vi "Compute Max Level.vi"(0 "FM Sweep in":refnum<class "FM Sweep.lvclass">, 1 "Filter in":refnum<class "Filter.lvclass">, 5 "Level in":refnum<class "Level.lvclass">, 7 "Fs (Hz)":dbl, 9 "Vmax":dbl, 11 "error in (no error)":errorcluster) -> (4 "FM Sweep out":refnum<class "FM Sweep.lvclass">, 6 "Level thru":refnum<class "Level.lvclass">, 10 "Lmax":dbl, 15 "error out":errorcluster)   [LabVIEW 2020, in "FM Sweep.lvclass"]
uses:
  FM Sweep.lvclass
  D:/Experiment VIs/Koop/KObject Class/KObject.lvclass
  Level/Level.lvclass
  Filter/Filter.lvclass
  FM Sweep.lvclass/FM Sweep.ctl
  Level/Level.lvclass/Level.ctl
  <vilib>/Analysis/baseanly.llb/Mean (DBL).vi
  Level/Read Units.vi
  Utility VIs/Math VIs/Linear to dB (scalar).vi
  <vilib>/Analysis/NI_AALBase.lvlib
  Koop/KObject Class/KObject.lvclass
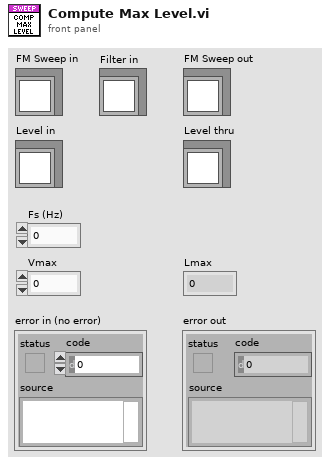
[diagram p1: front panel]
types:
  T1 = typedef "Level.lvclass/LevelUnits.ctl" = enum16{"dB atten", "dB SPL", "dB Vrms", "Volts", "dB mW", "mW", "dB HL", "dB SL"}
  T2 = cluster{"Freq (Hz)":dbl[], "Mag (dB SPL)":dbl[], "Phase (deg)":dbl[]}
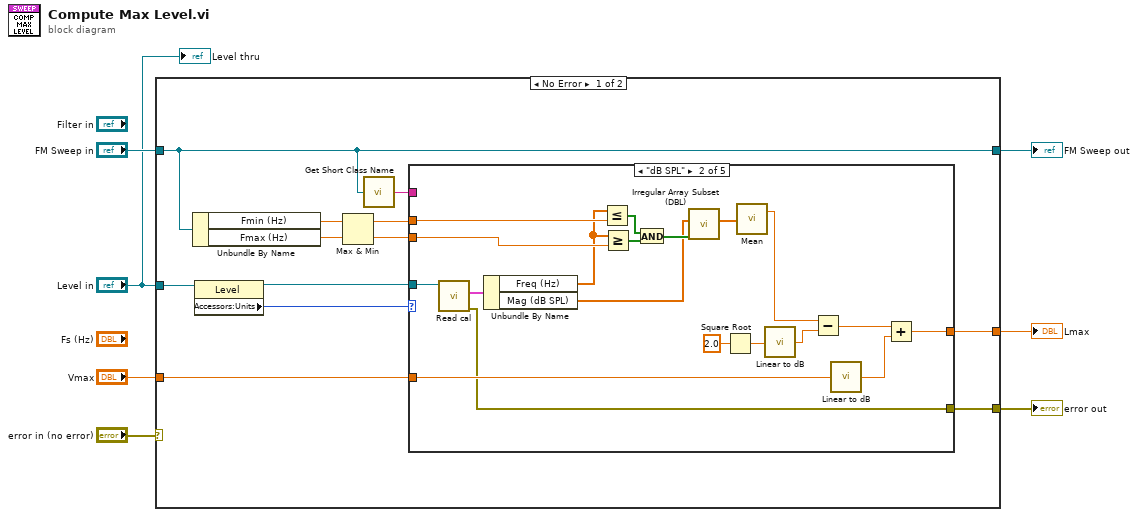
[diagram p0: block diagram]
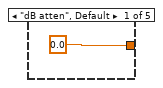
[diagram p2: hidden frame]
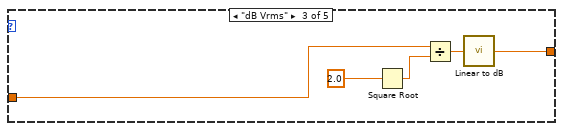
[diagram p3: hidden frame]
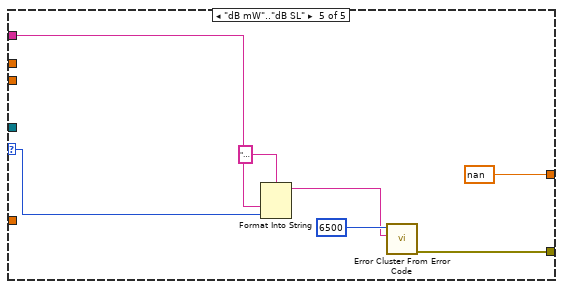
[diagram p5: hidden frame]
diagram:
  n1 = case shown="No Error" "error in (no error)" {
    selector: "error in (no error)" -> [_ w53]
    tunnel: "FM Sweep in" -> [w14 w54]
    tunnel: [w14 w54] -> w6
    tunnel: "Level in" -> [w19 _]
    tunnel: "Vmax" -> [w17 _]
    tunnel: [w16 _] -> w3
    tunnel: [w15 w53] -> w2
    frame No Error {
      n2 = Unbundle By Name(w14) -> ("Fmin (Hz)"=w11:dbl, "Fmax (Hz)"=w10:dbl)
      n3 = property class="Level"(reference=w19) -> (reference out=w12:refnum<class "Level.lvclass">, "Accessors:Units"=w18:T1)  [unwired: 1 in, 1 out]
      n4 = Max & Min(x=w11, y=w10) -> (max(x,y)=w9:dbl, min(x,y)=w8:dbl)
      n5 = call "Get Short Class Name.vi"("KObject in"=w14) -> ("Class"=w13:string)  [unwired: 4 in]
      n6 = case shown="\"dB SPL\"" w18 {
        selector: w18 -> [_ _ _ _ w47]
        tunnel: [0.0 ("Reference Level") w39 w41 w45 nan ("Vmax")] -> w16
        tunnel: [_ w21 _ _ w49] -> w15
        tunnel: w9 -> [_ w28 _ _ _]
        tunnel: w8 -> [_ w27 _ _ _]
        tunnel: w17 -> [_ w26 w40 w45 _]
        tunnel: w13 -> [_ _ _ _ w46]
        tunnel: w12 -> [_ w25 _ _ _]
        frame "dB atten", Default {
        }
        frame "dB SPL" {
          n7 = call "Read cal.vi"("Level in"=w25) -> ("error out"=w21:errorcluster, "cal"=w24:T2)  [unwired: 8 in, 1 out]
          n8 = Unbundle By Name(w24) -> ("Freq (Hz)"=w23:dbl[], "Mag (dB SPL)"=w22:dbl[])
          n9 = Less Or Equal?(x=w23, y=w28) -> (x <= y?=w33:bool[])
          n10 = Greater Or Equal?(x=w23, y=w27) -> (x >= y?=w32:bool[])
          n11 = And(x=w33, y=w32) -> (x .and. y?=w31:bool[])
          n12 = call "Irregular Array Subset (DBL).vi"("Mask"=w31, "Array"=w22) -> ("Array Subset"=w30:dbl[])  [unwired: 8 in, 1 out]
          n13 = Square Root(x=2.0 ("y")) -> (sqrt(x)=w36:dbl)
          n14 = call-poly <vilib>:"Mean.vi"("X"=w30) -> ("mean"=w29:dbl)  [unwired: 1 out]
          n15 = call-poly "Linear to dB.vi"("Linear"=w36) -> ("dB"=w35:dbl)
          n16 = Subtract(x=w29, y=w35) -> (x-y=w34:dbl)
          n17 = call-poly "Linear to dB.vi"("Linear"=w26) -> ("dB"=w38:dbl)
          n18 = Add(x=w34, y=w38) -> (x+y=w39:dbl)
        }
        frame "dB Vrms" {
          n19 = Square Root(x=2.0 ("y")) -> (sqrt(x)=w43:dbl)
          n20 = Divide(x=w40, y=w43) -> (x/y=w42:dbl)
          n21 = call-poly "Linear to dB.vi"("Linear"=w42) -> ("dB"=w41:dbl)
        }
        frame "Volts" {
        }
        frame "dB mW".."dB SL" {
          n22 = Format Into String(format string="%s: Cannot set level in '%s'", w46, w47) -> (resulting string=w50:string)  [unwired: 2 in, 1 out]
          n23 = call <vilib>:"Error Cluster From Error Code.vi"("error message (\"\")"=w50, "error code (0)"=6500) -> ("error out"=w49:errorcluster)  [unwired: 7 in]
        }
      }
    }
    frame Error {
    }
  }
  "error out" <- w2
  "FM Sweep out" <- w6
  "Lmax" <- w3
  "Level thru" <- "Level in"
